vi "Get Outline.vi"(6 "Scale Factor":i32=1, 8 "error in (no error)":errorcluster, 9 "Y Offset":i32, 10 "X Offset":i32, 11 "Outline in":refnum<class "Outline.lvclass">) -> (0 "error out":errorcluster, 2 "Outline":cluster{"X":i32, "Y":i32}[](array[cluster]), 3 "Outline out":refnum<class "Outline.lvclass">)   [LabVIEW 2013, in "Outline.lvclass"]
uses:
  Outline.lvclass
  Outline.lvclass/Outline.ctl
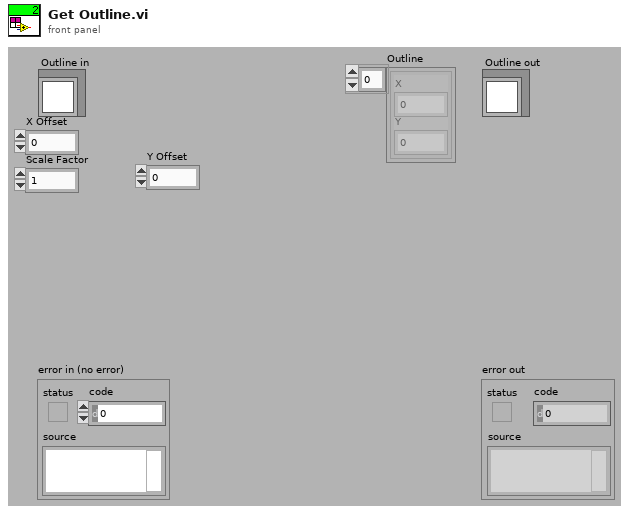
[diagram p1: front panel]
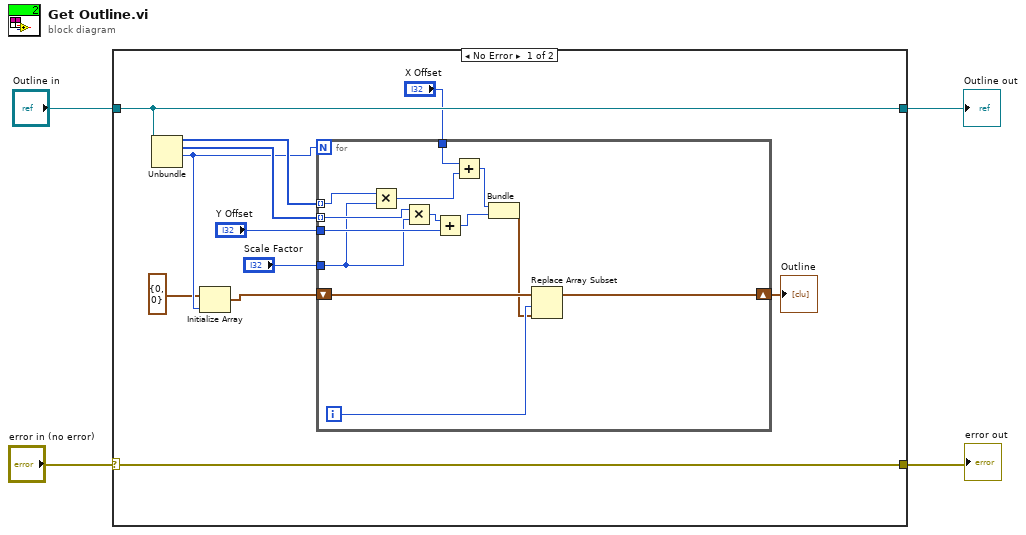
[diagram p0: block diagram]
diagram:
  n1 = case shown="No Error" "error in (no error)" {
    selector: "error in (no error)" -> [w15 w30]
    tunnel: [w15 w30] -> w3
    tunnel: [w14 w29] -> w1
    tunnel: "Outline in" -> [w14 w29]
    frame No Error {
      n2 = Unbundle(w14) -> (w13:i32[], w12:i32[], w11:i32)  [unwired: 1 out]
      n3 = Initialize Array(cluster{"X":i32, "Y":i32} {"X"=0, "Y"=0} ("Point Coordinates"), w11) -> (w9:cluster{"X":i32, "Y":i32}[])
      n4 = for {
        N: w11 -> [_]
        tunnel: w13 -> [w20] mode=indexing
        tunnel: w12 -> [w18] mode=indexing
        shift-right: [w26] -> w8
        shift-left: w9 -> [w27]
        tunnel: "X Offset" -> [w24]
        tunnel: "Y Offset" -> [w22]
        tunnel: "Scale Factor" -> [w17]
        i -> [w28]
        n5 = Multiply(x=w20, y=w17) -> (x*y=w19:i32)
        n6 = Multiply(x=w18, y=w17) -> (x*y=w16:i32)
        n7 = Add(x=w16, y=w22) -> (x+y=w21:i32)
        n8 = Add(x=w24, y=w19) -> (x+y=w23:i32)
        n9 = Bundle(w23, w21) -> (w25:cluster{i32, i32})  [unwired: 1 in]
        n10 = Replace Array Subset(array=w27, new element=w25, index=w28) -> (w26:cluster{"X":i32, "Y":i32}[])
      }
      "Outline" <- w8
    }
    frame Error {
    }
  }
  "error out" <- w3
  "Outline out" <- w1
